vi "Write Motor Data.vi"(8 "error in (no error)":errorcluster, 9 "Motor Data":T1, 10 "Motor":T2, 11 "MCB Status in":refnum<class "MCB Status.lvclass">) -> (0 "error out":errorcluster, 3 "MCB Status out":refnum<class "MCB Status.lvclass">)   [LabVIEW 2015, in "RDS Child Messages.lvlib" / "MCB Status.lvclass"]
uses:
  MCB Status.lvclass
  MCB Channel.ctl
  MCB Motor Status.ctl
  MCB Status.lvclass/MCB Status.ctl
  RDS Child Messages.lvlib
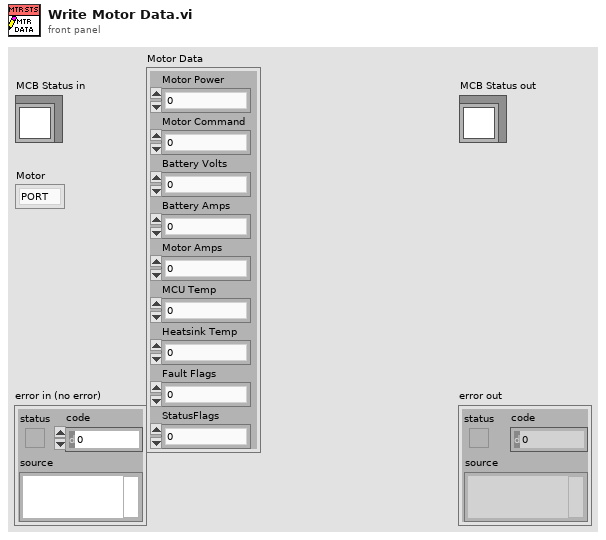
[diagram p1: front panel]
types:
  T1 = typedef "RDS Child Messages.lvlib/MCB Motor Status.ctl" = cluster{"Motor Power":i16, "Motor Command":i16, "Battery Volts":sgl, "Battery Amps":sgl, "Motor Amps":sgl, "MCU Temp":i16, "Heatsink Temp":i16, "Fault Flags":u16, "StatusFlags":u16}
  T2 = typedef "RDS Child Messages.lvlib/MCB Channel.ctl" = enum16{"PORT", "STBD"}
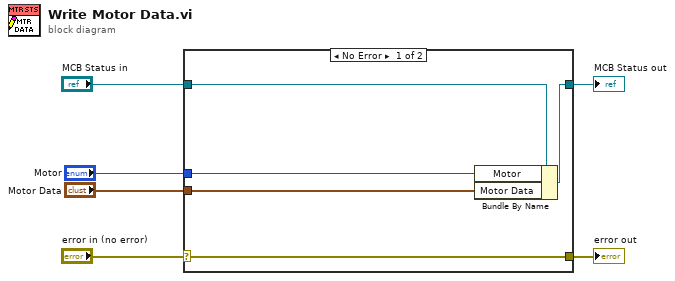
[diagram p0: block diagram]
diagram:
  n1 = case shown="No Error" "error in (no error)" {
    selector: "error in (no error)" -> [w11 w12]
    tunnel: [w11 w12] -> w5
    tunnel: [w9 w13] -> w3
    tunnel: "MCB Status in" -> [w10 w13]
    tunnel: "Motor" -> [w8 _]
    tunnel: "Motor Data" -> [w7 _]
    frame No Error {
      n2 = Bundle By Name(cluster=w10, "Motor"=w8, "Motor Data"=w7) -> (w9:refnum<class "MCB Status.lvclass">)
    }
    frame Error {
    }
  }
  "error out" <- w5
  "MCB Status out" <- w3
